vi "get stable RF voltage.vi"(9 "diode steady state voltage":dbl) -> (1 "stable voltage":dbl, 2 "polarimeter task out":refnum<k21>, 3 "rf gen task out":refnum<k21>)   [LabVIEW 2018]
uses:
  <vilib>/DAQmx/write.llb/DAQmx Write (Analog DBL 1Chan 1Samp).vi
  4f967cfa-f295-4c21-8527-c71cc98837c5.vi
  f9da4950-4a72-4538-adda-a8c4b27a076f.vi
  <vilib>/DAQmx/read.llb/DAQmx Read (Analog DBL 1Chan 1Samp).vi
  <vilib>/DAQmx/create/channels.llb/DAQmx Create Channel (AO-Voltage-Basic).vi
  <vilib>/DAQmx/create/channels.llb/DAQmx Create Channel (AI-Voltage-Basic).vi
  <vilib>/DAQmx/miscellaneous.llb/DAQmx Fill In Error Info.vi
panel:
  in  "diode channel":tag
  in  "rf gen channel":tag
  in  "start voltage":dbl=0.3 format="%#_13g"
  out "Waveform Chart":dbl(graph)
  out "current rf voltage in":dbl
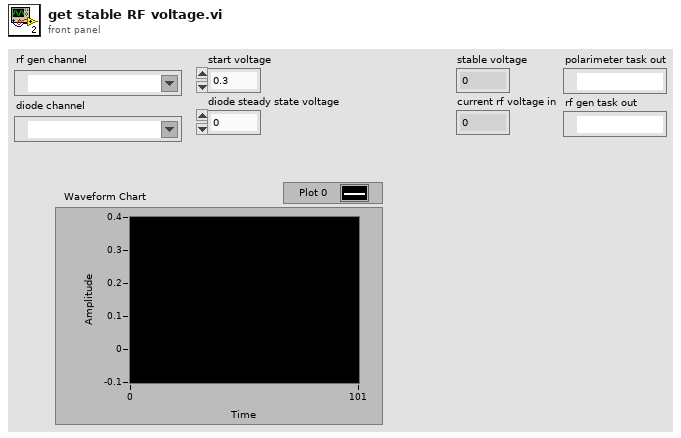
[diagram p1: front panel]
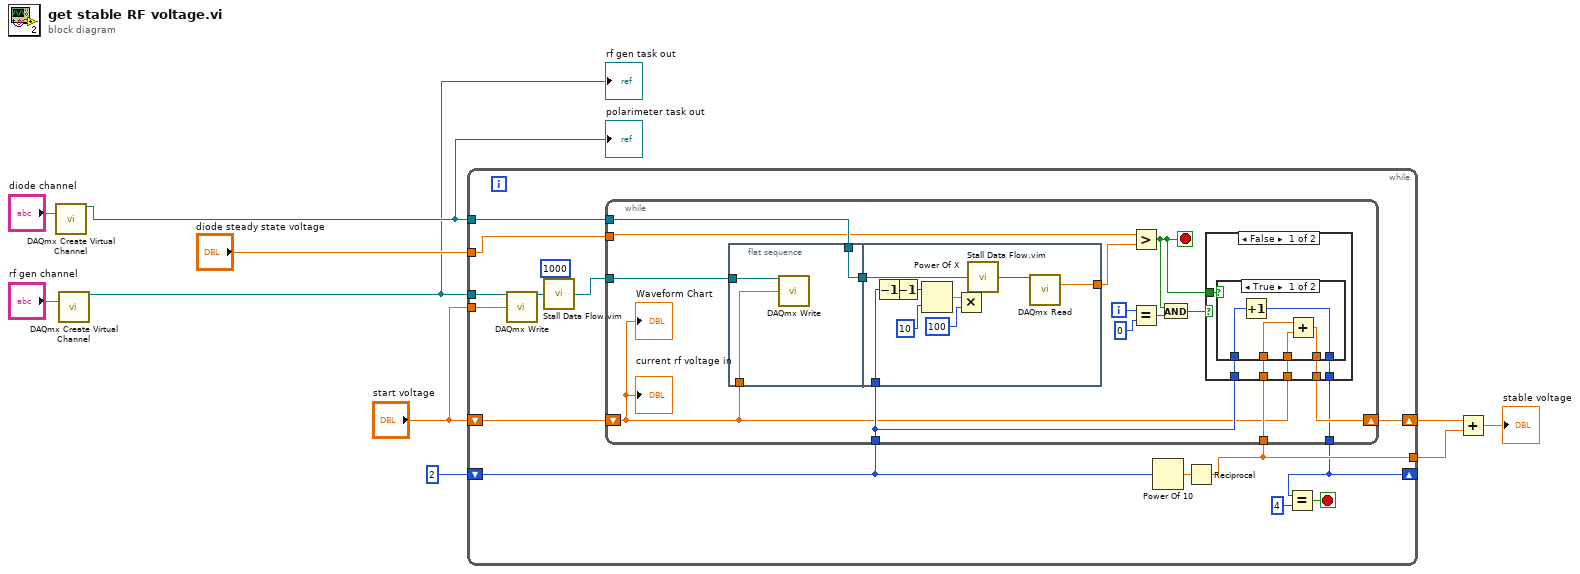
[diagram p0: block diagram]
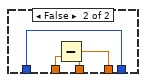
[diagram p2: hidden frame]
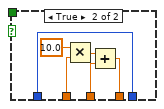
[diagram p3: hidden frame]
diagram:
  n1 = call-poly <vilib>:"DAQmx Create Virtual Channel.vi"("physical channels"="diode channel") -> ("task out"=w2:refnum<k21>)  [unwired: 13 in, 1 out]
  "polarimeter task out" <- w2
  n2 = call-poly <vilib>:"DAQmx Create Virtual Channel.vi"("physical channels"="rf gen channel") -> ("task out"=w1:refnum<k21>)  [unwired: 13 in, 1 out]
  "rf gen task out" <- w1
  n3 = while {
    tunnel: w2 -> [w14]
    shift-right: [w18] -> w6
    shift-left: "start voltage" -> [w11]
    tunnel: w1 -> [w22]
    tunnel: "start voltage" -> [w21]
    shift-right: [w15] -> _
    shift-left: 2 -> [w17]
    tunnel: [w16] -> w8
    tunnel: "diode steady state voltage" -> [w12]
    stop <- w19 stop-if-true
    n4 = call-poly <vilib>:"DAQmx Write.vi"("task/channels in"=w22, "data"=w21) -> ("task out"=w24:refnum<k21>)  [unwired: 11 in, 2 out]
    n5 = call "Stall Data Flow.vim"("value in"=w24, "milliseconds to wait"=u32 1000) -> ("value out"=w13:refnum<k21>)  [unwired: 1 out]
    n6 = Power Of 10(x=w17) -> (10^x=w25:dbl)
    n7 = Reciprocal(x=w25) -> (1/x=w16:dbl)
    n8 = while {
      tunnel: w14 -> [w32]
      tunnel: w13 -> [w33]
      shift-right: [w35] -> w18
      shift-left: w11 -> [w27]
      tunnel: w16 -> [w36]
      tunnel: w17 -> [w30]
      tunnel: [w34] -> w15
      tunnel: w12 -> [w26]
      i -> [w40]
      stop <- w28 stop-if-true
      n9 = flat-sequence {
        tunnel: w27 -> [w43]
        tunnel: w33 -> [w42]
        tunnel: w32 -> [w41]
        tunnel: [w41] -> w31
        tunnel: w31 -> [w46]
        tunnel: w30 -> [w45]
        tunnel: [w44] -> w29
        frame #0 {
          n10 = call-poly <vilib>:"DAQmx Write.vi"("task/channels in"=w42, "data"=w43) -> ()  [unwired: 11 in, 3 out]
        }
        frame #1 {
          n11 = Decrement(x=w45) -> (x-1=w51:i32)
          n12 = Decrement(x=w51) -> (x-1=w47:i32)
          n13 = Power Of X(1:10 ("y"), 2:w47) -> (0:w48:dbl)
          n14 = Multiply(x=w48, y=100) -> (x*y=w49:dbl)
          n15 = call "Stall Data Flow.vim"("value in"=w46, "milliseconds to wait"=w49) -> ("value out"=w53:refnum<k21>)  [unwired: 1 out]
          n16 = call-poly <vilib>:"DAQmx Read.vi"("task/channels in"=w53) -> ("data"=w44:dbl)  [unwired: 12 in, 2 out]
        }
      }
      n17 = Greater?(x=w26, y=w29) -> (0:w28:bool)
      n18 = Equal?(x=w40, y=0) -> (x = y?=w38:bool)
      n19 = And(x=w28, y=w38) -> (x .and. y?=w37:bool)
      n20 = case shown="False" w37 {
        tunnel: w36 -> [w57 w74]
        tunnel: w27 -> [w58 w71]
        tunnel: [w59 w70] -> w35
        tunnel: w30 -> [w56 w69]
        tunnel: [w55 w69] -> w34
        tunnel: w28 -> [w54 _]
        frame False {
          n21 = case shown="True" w54 {
            tunnel: [w64 w66] -> w59
            tunnel: w58 -> [w63 w68]
            tunnel: w57 -> [w62 w67]
            tunnel: w56 -> [w61 w65]
            tunnel: [w60 w65] -> w55
            frame True {
              n22 = Increment(x=w61) -> (x+1=w60:i32)
              n23 = Add(x=w62, y=w63) -> (x+y=w64:dbl)
            }
            frame False {
              n24 = Subtract(x=w68, y=w67) -> (x-y=w66:dbl)
            }
          }
        }
        frame True {
          n25 = Multiply(x=10.0, y=w74) -> (x*y=w72:dbl)
          n26 = Add(x=w72, y=w71) -> (x+y=w70:dbl)
        }
      }
      "Waveform Chart" <- w27
      "current rf voltage in" <- w27
    }
    n27 = Equal?(x=w15, y=4) -> (x = y?=w19:bool)
  }
  n28 = Add(x=w6, y=w8) -> (x+y=→"stable voltage":dbl)
